vi "Loan.vi"() -> ()   [LabVIEW 2009]
panel:
  out "Monthly Installment":dbl
  in  "Rate of Interest (%)":dbl
  in  "Time (Year)":dbl
  in  "Loan Amount":dbl
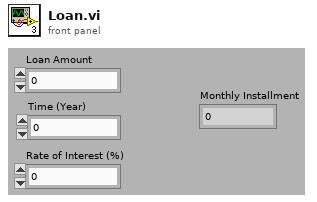
[diagram p1: front panel]
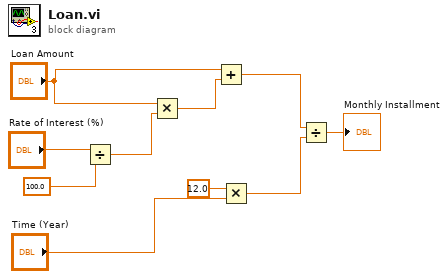
[diagram p0: block diagram]
diagram:
  n1 = Divide(x="Rate of Interest (%)", y=100.0) -> (x/y=w8:dbl)
  n2 = Multiply(x="Loan Amount", y=w8) -> (x*y=w6:dbl)
  n3 = Add(x="Loan Amount", y=w6) -> (x+y=w3:dbl)
  n4 = Multiply(x=12.0, y="Time (Year)") -> (x*y=w2:dbl)
  n5 = Divide(x=w3, y=w2) -> (x/y=→"Monthly Installment":dbl)
